vi "waveformGraphInputs.vi"() -> ()   [LabVIEW 2014]
panel:
  in  "Step Size":dbl(slide)=0.5 scale=0.0..3.0
  in  "Start Value":dbl(slide)=20.0 scale=0.0..50.0
  out "Multiple Heterogeneous Sample Waveform Graph 2\n(X-Values supplied as Heterogeneous Start Value and Step Size)":cluster{dbl, dbl, dbl[]}[](graph)
  out "Multiple Heterogeneous Sample Waveform Graph 2\n(X-Values supplied as Start Value and Step Size)":T1(graph)
  out "Multiple Heterogeneous Sample Waveform Graph 1\n(Array Index Used as X-value)":cluster{dbl[]}[](graph)
  out "Multiple  Homogeneous Sample Waveform Graph 2\n(X-Values supplied as Start Value and Step Size)":T2(graph)
  out "Multiple Homogeneous Sample Waveform Graph 1\n(Array Index Used as X-value)":dbl[][](graph)
  out "Single Sample Waveform Graph 3\n(Data Supplied as \"Waveform\" Type)":waveform(dbl)(graph)
  out "Single Sample Waveform Graph 2\n(X-Values supplied as Start Value and Step Size)":T3(graph)
  out "Single Sample Waveform Graph 1\n(Array Index Used as X-value)":dbl[](graph)
  # "Sampling Controls"
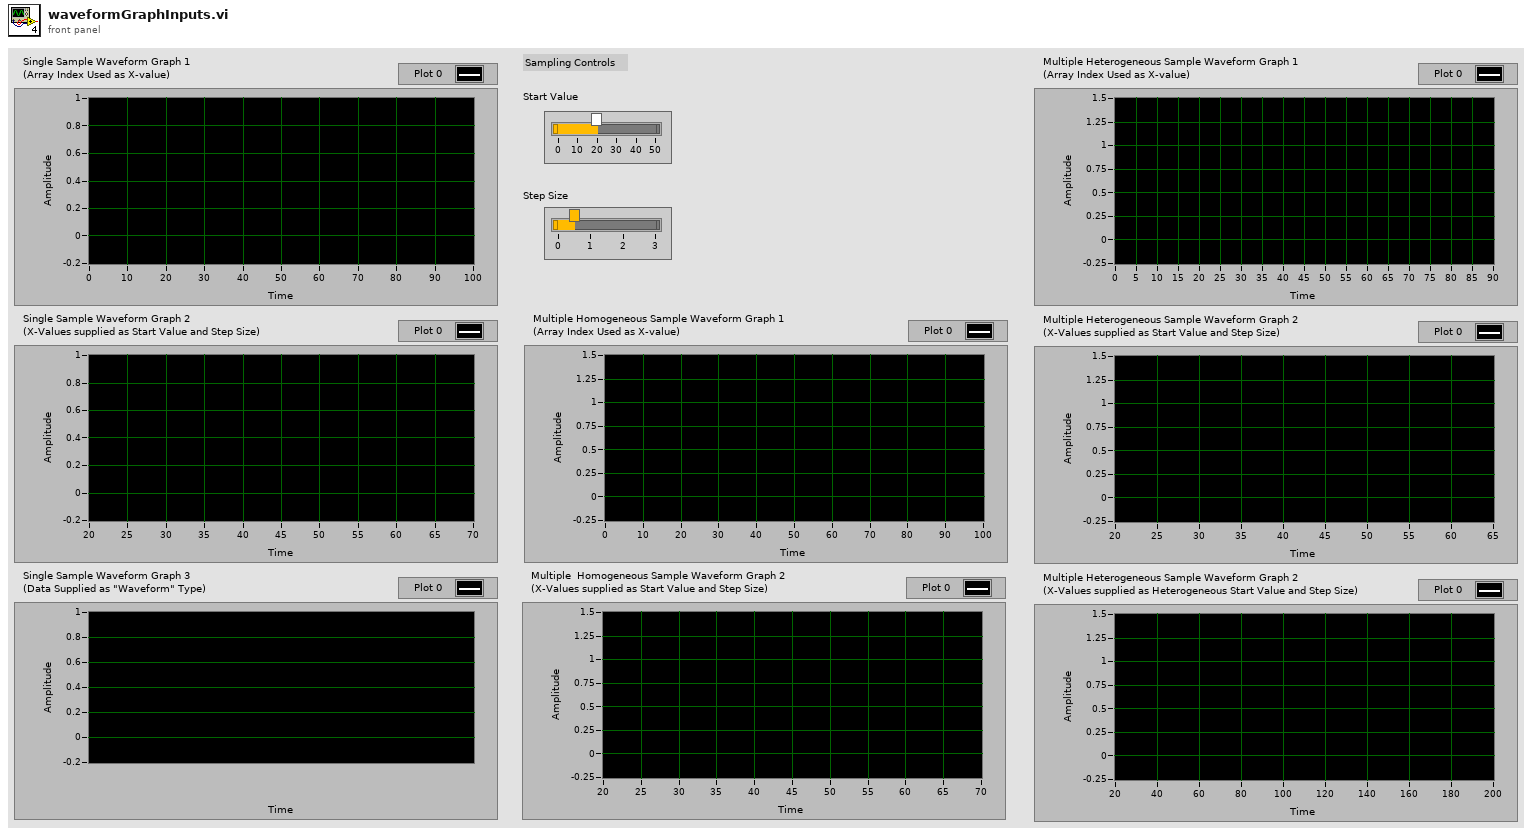
[diagram p1: front panel]
types:
  T1 = cluster{"Start Value":dbl, "Step Size":dbl, cluster{dbl[]}[]}
  T2 = cluster{"Start Value":dbl, "Step Size":dbl, dbl[][]}
  T3 = cluster{"Start Value":dbl, "Step Size":dbl, dbl[]}
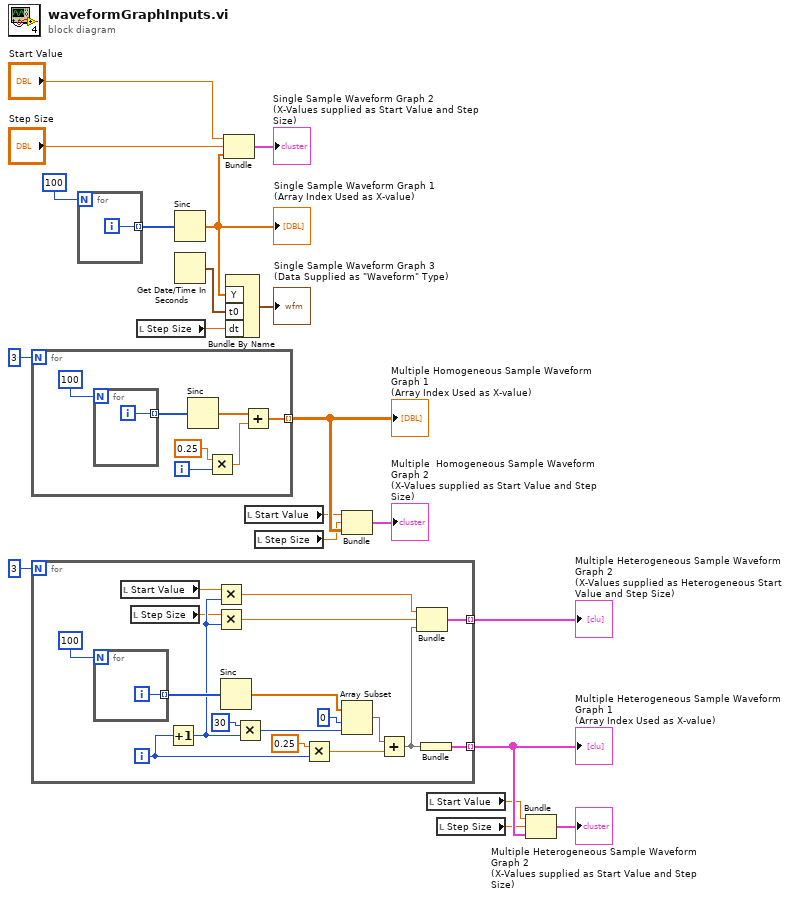
[diagram p0: block diagram]
diagram:
  n1 = for {
    N: 3 -> [_]
    tunnel: [w24] -> w12 mode=indexing
    i -> [w23]
    n2 = for {
      N: 100 -> [_]
      tunnel: [w28] -> w27 mode=indexing
      i -> [w28]
    }
    n3 = Sinc(1:w27) -> (0:w25:dbl[])
    n4 = Multiply(x=0.25, y=w23) -> (x*y=w22:dbl)
    n5 = Add(x=w25, y=w22) -> (x+y=w24:dbl[])
  }
  "Multiple Homogeneous Sample Waveform Graph 1\n(Array Index Used as X-value)" <- w12
  n6 = for {
    N: 3 -> [_]
    tunnel: [w33] -> w10 mode=indexing
    tunnel: [w32] -> w8 mode=indexing
    i -> [w37]
    n7 = for {
      N: 100 -> [_]
      tunnel: [w47] -> w46 mode=indexing
      i -> [w47]
    }
    n8 = local read "Start Value"() -> (w30:dbl)
    n9 = local read "Step Size"() -> (w29:dbl)
    n10 = Increment(x=w37) -> (x+1=w35:i32)
    n11 = Multiply(x=w30, y=w35) -> (x*y=w34:dbl)
    n12 = Multiply(x=w29, y=w35) -> (x*y=w36:dbl)
    n13 = Sinc(1:w46) -> (0:w42:dbl[])
    n14 = Multiply(x=30, y=w35) -> (x*y=w39:i32)
    n15 = Multiply(x=0.25, y=w37) -> (x*y=w44:dbl)
    n16 = Array Subset(array=w42, index=0, length=w39) -> (w38:dbl[])
    n17 = Add(x=w38, y=w44) -> (x+y=w31:dbl[])
    n18 = Bundle "Bundle"(w34, w36, w31) -> (w32:cluster{dbl, dbl, dbl[]})  [unwired: 1 in]
    n19 = Bundle "Bundle"(w31) -> (w33:cluster{dbl[]})  [unwired: 1 in]
  }
  "Multiple Heterogeneous Sample Waveform Graph 1\n(Array Index Used as X-value)" <- w10
  "Multiple Heterogeneous Sample Waveform Graph 2\n(X-Values supplied as Heterogeneous Start Value and Step Size)" <- w8
  n20 = for {
    N: 100 -> [_]
    tunnel: [w48] -> w20 mode=indexing
    i -> [w48]
  }
  n21 = local read "Step Size"() -> (w7:dbl)
  n22 = Sinc(1:w20) -> (0:w17:dbl[])
  "Single Sample Waveform Graph 1\n(Array Index Used as X-value)" <- w17
  n23 = Get Date/Time In Seconds() -> (seconds since 1Jan1904=w15:timestamp)
  n24 = Bundle "Bundle"("Start Value"="Start Value", "Step Size"="Step Size", w17) -> (→"Single Sample Waveform Graph 2\n(X-Values supplied as Start Value and Step Size)":T3)  [unwired: 1 in]
  n25 = Bundle By Name("Y"=w17, "t0"=w15, "dt"=w7) -> (→"Single Sample Waveform Graph 3\n(Data Supplied as \"Waveform\" Type)":waveform(dbl))  [unwired: 1 in]
  n26 = local read "Start Value"() -> (w6:dbl)
  n27 = local read "Step Size"() -> (w3:dbl)
  n28 = Bundle "Bundle"("Start Value"=w6, "Step Size"=w3, w12) -> (→"Multiple  Homogeneous Sample Waveform Graph 2\n(X-Values supplied as Start Value and Step Size)":T2)  [unwired: 1 in]
  n29 = local read "Start Value"() -> (w5:dbl)
  n30 = local read "Step Size"() -> (w4:dbl)
  n31 = Bundle "Bundle"("Start Value"=w5, "Step Size"=w4, w10) -> (→"Multiple Heterogeneous Sample Waveform Graph 2\n(X-Values supplied as Start Value and Step Size)":T1)  [unwired: 1 in]
